vi "Set IC.vi"(8 "error in (no error)":errorcluster, 10 "IC":variant, 11 "IC_1D_VIRef in":refnum<class "NI_IC_1D_VIRef.lvclass">) -> (0 "error out":errorcluster, 3 "IC_1D_VIRef out":refnum<class "NI_IC_1D_VIRef.lvclass">)   [LabVIEW 2020, in "NI_PDE.lvlib" / "NI_IC_1D_VIRef.lvclass"]
uses:
  <vilib>/gmath/pde.llb/ICClass/IC_1D_VIRef/NI_IC_1D_VIRef.lvclass
  <vilib>/gmath/pde.llb/ICClass/IC_1D_VIRef/IC Data.ctl
  <vilib>/gmath/pde.llb/Common/PDE_IC Type.ctl
  <vilib>/gmath/pde.llb/ICClass/IC_1D_VIRef/NI_IC_1D_VIRef.lvclass/NI_IC_1D_VIRef.ctl
  <vilib>/gmath/NI_PDE.lvlib
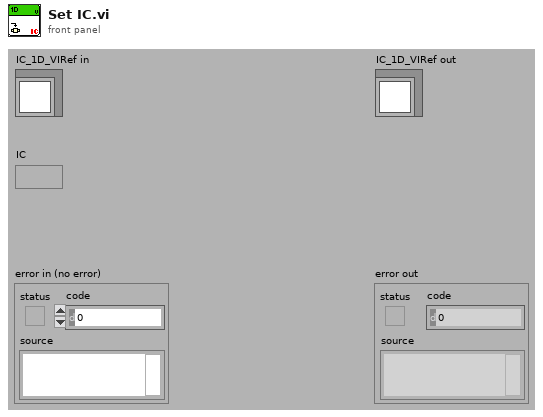
[diagram p1: front panel]
types:
  T1 = typedef "NI_PDE.lvlib/NI_IC_1D_VIRef.lvclass/IC Data.ctl" = cluster{"type":T2, "H":refnum<vi>, "data":variant}
  T2 = typedef "NI_PDE.lvlib/PDE_IC Type.ctl" = i32
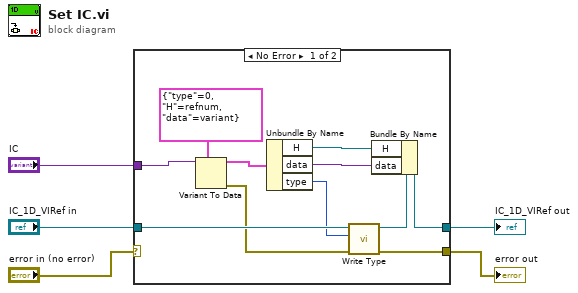
[diagram p0: block diagram]
diagram:
  n1 = case shown="No Error" "error in (no error)" {
    selector: "error in (no error)" -> [_ w18]
    tunnel: "IC_1D_VIRef in" -> [w14 w17]
    tunnel: [w10 w17] -> w5
    tunnel: [w9 w18] -> w4
    tunnel: "IC" -> [w15 _]
    frame No Error {
      n2 = Variant To Data(type=T1 {"type"=0, "H"=refnum, "data"=variant} ("IC data"), Variant=w15) -> (data=w13:T1, error out=w12:errorcluster)  [unwired: 1 in]
      n3 = Unbundle By Name(w13) -> ("H"=w8:refnum<vi>, "data"=w7:variant, "type"=w6:T2)
      n4 = call-dynamic "Write Type.vi"("error in (no error)"=w12, "IC type"=w6, "IC.lvclass in"=w14) -> ("error out"=w9:errorcluster, "IC.lvclass out"=w11:refnum<class "NI_IC_1D_VIRef.lvclass">)  [unwired: 7 out]
      n5 = Bundle By Name(cluster=w11, "H"=w8, "data"=w7) -> (w10:refnum<class "NI_IC_1D_VIRef.lvclass">)
    }
    frame Error {
    }
  }
  "IC_1D_VIRef out" <- w5
  "error out" <- w4
